vi "PS Replace NaN with Zero.vi"(7 "Input waveform":waveform(dbl)) -> (8 "Output waveform":waveform(dbl))   [LabVIEW 2021, in "DAQ_Power Supply Source and Measure.lvlib"]
doc: "This VI takes a single waveform as input and replaces all NaN values with zeros and returned the modified waveform as output"
uses:
  DAQ_Power Supply Source and Measure.lvlib
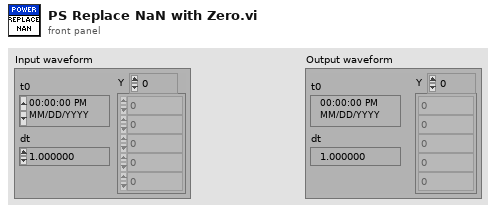
[diagram p1: front panel]
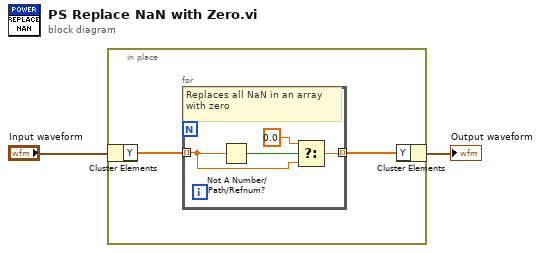
[diagram p0: block diagram]
diagram:
  n1 = in-place {
    n2 = in-place-cluster #1("Input waveform") -> ("Y"=w4:dbl[])
    n3 = for {
      tunnel: w4 -> [w6] mode=indexing
      tunnel: [w5] -> w3 mode=indexing
      # "Replaces all NaN in an array with zero"
      n4 = Not A Number/Path/Refnum?(number/path/refnum=w6) -> (NaN/Path/Refnum?=w8:bool)
      n5 = Select(t=0.0, s=w8, f=w6) -> (s? t:f=w5:dbl)
    }
    n6 = in-place-cluster #1("Y"=w3) -> (→"Output waveform":waveform(dbl))
  }
